vi "rotHexPos.vi"(7 "Tilt Angle (arcsec)":cluster{"Tile X":dbl, "Tilt Y":dbl}, 8 "error in (no error)":errorcluster, 9 "Hexapod DOF":dbl[](array[numeric]), 10 "Hexapod":enum16{"Camera", "M2"}(ring), 11 "CamRot in":refnum<class "CamRot.lvclass">) -> (0 "error out":errorcluster, 2 "Rotated Hexapod DOF":dbl[](array[numeric]), 3 "CamRot out":refnum<class "CamRot.lvclass">)   [LabVIEW 2016, in "OfcFunc.lvlib" / "CamRot.lvclass"]
doc: "Rotate the hexapod position (degree of freedom, DOF) based on the rotation angle."
uses:
  CamRot.lvclass
  CamRot.lvclass/CamRot.ctl
  MatOper/MatOper.lvclass
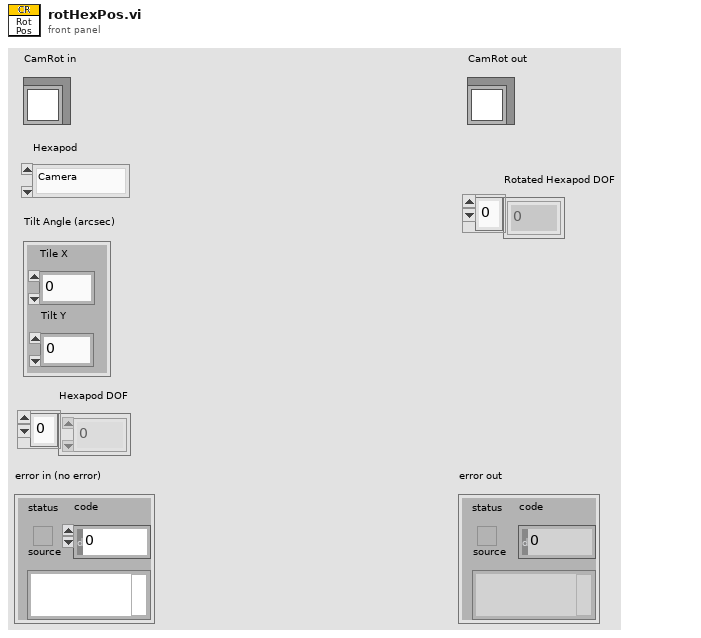
[diagram p1: front panel]
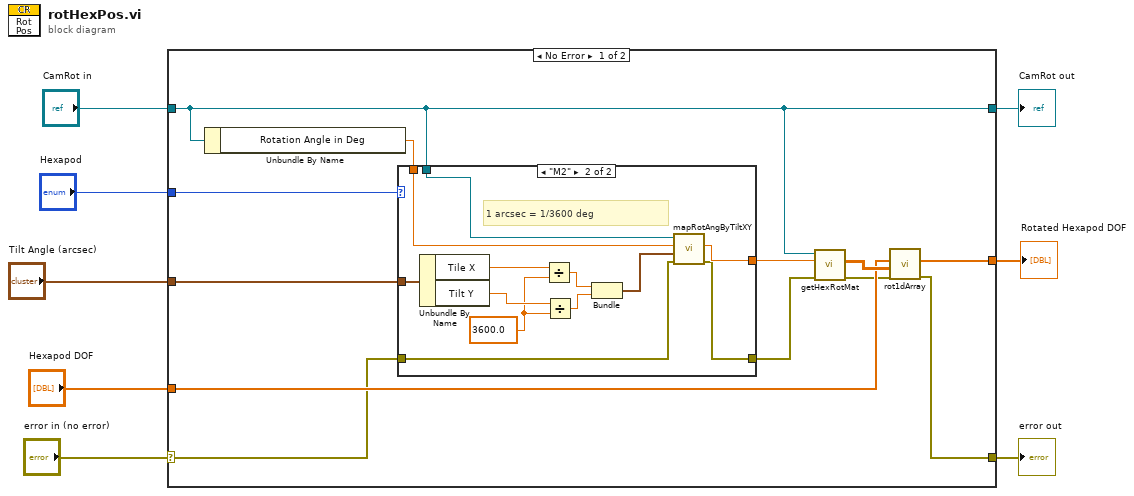
[diagram p0: block diagram]
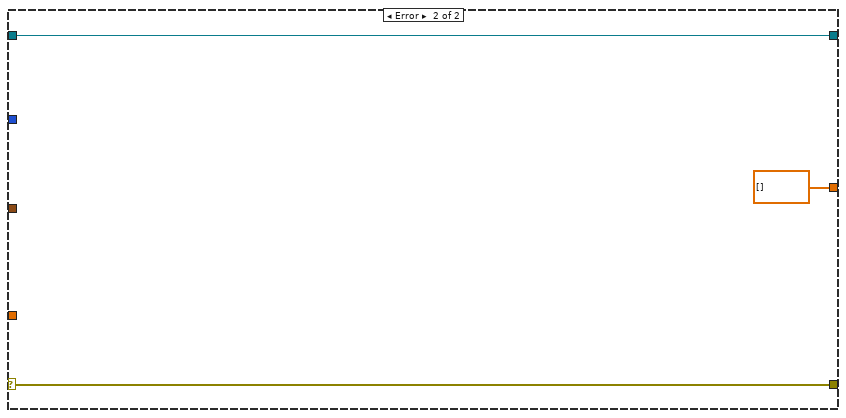
[diagram p3: hidden frame]
diagram:
  n1 = case shown="No Error" "error in (no error)" {
    selector: "error in (no error)" -> [w13 w37]
    tunnel: [w12 w37] -> w7
    tunnel: [w17 w36] -> w5
    tunnel: "CamRot in" -> [w17 w36]
    tunnel: "Hexapod" -> [w19 _]
    tunnel: "Tilt Angle (arcsec)" -> [w18 _]
    tunnel: "Hexapod DOF" -> [w14 _]
    tunnel: [w9 dbl[] [] ("Rotated 1D Array")] -> w1
    frame No Error {
      n2 = Unbundle By Name(w17) -> ("Rotation Angle in Deg"=w20:dbl)
      n3 = case shown="\"M2\"" w19 {
        tunnel: w20 -> [w22 w27]
        tunnel: [w22 w25] -> w16
        tunnel: w17 -> [_ w28]
        tunnel: w18 -> [_ w34]
        tunnel: w13 -> [w21 w24]
        tunnel: [w21 w23] -> w11
        frame "Camera", Default {
        }
        frame "M2" {
          w31 = 3600.0
          # "1 arcsec = 1/3600 deg"
          n4 = Unbundle By Name(w34) -> ("Tile X"=w33:dbl, "Tilt Y"=w32:dbl)
          n5 = Divide(x=w33, y=w31) -> (x/y=w30:dbl)
          n6 = Divide(x=w32, y=w31) -> (x/y=w29:dbl)
          n7 = Bundle(w30, w29) -> (w26:cluster{dbl, dbl})  [unwired: 1 in]
          n8 = call "mapRotAngByTiltXY.vi"("error in (no error)"=w24, "Tilt Angle (degree)"=w26, "Rotation Angle in Deg"=w27, "CamRot in"=w28) -> ("error out"=w23:errorcluster, "Mapped Rotation Angle in Deg"=w25:dbl)  [unwired: 5 in, 1 out]
        }
      }
      n9 = call "getHexRotMat.vi"("error in (no error)"=w11, "Rotation Angle in Deg"=w16, "CamRot in"=w17) -> ("error out"=w10:errorcluster, "Rotation Matrix"=w15:dbl[][])  [unwired: 6 in, 1 out]
      n10 = call "rot1dArray.vi"("error in (no error)"=w10, "Rot Mat"=w15, "1D Array"=w14) -> ("error out"=w12:errorcluster, "Rotated 1D Array"=w9:dbl[])  [unwired: 6 in, 1 out]
    }
    frame Error {
    }
  }
  "error out" <- w7
  "CamRot out" <- w5
  "Rotated Hexapod DOF" <- w1
